vi "getOutputStateArray.vi"(8 "error in (no error)":errorcluster, 10 "configuration_name":string, 11 "HWConfiguration in":refnum<class "HWConfigurations.lvclass">) -> (0 "error out":errorcluster, 2 "outputStateArray":cluster{"channel":string, "state":string}[](array[cluster]), 3 "HWConfiguration out":refnum<class "HWConfigurations.lvclass">)   [LabVIEW 2009, in "Tools.lvlib" / "DatabaseHelpers.lvlib" / "HWConfigurations.lvclass"]
uses:
  HWConfigurations.lvclass
  HWConfigurations.lvclass/HWConfigurations.ctl
  OutputConfiguration/OutputConfiguration.lvclass
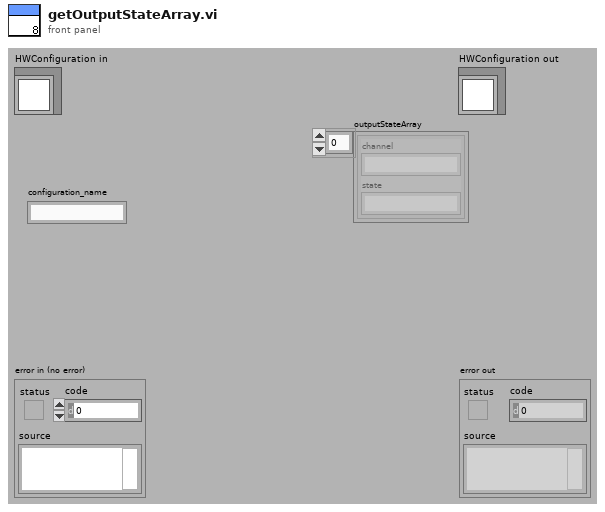
[diagram p1: front panel]
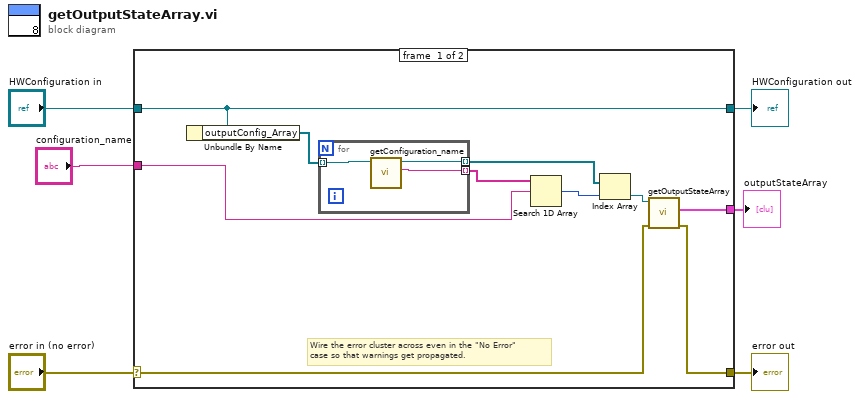
[diagram p0: block diagram]
diagram:
  n1 = case shown="No Error" "error in (no error)" {
    selector: "error in (no error)" -> [w9 w21]
    tunnel: [w8 w21] -> w5
    tunnel: [w16 w20] -> w3
    tunnel: "HWConfiguration in" -> [w16 w20]
    tunnel: "configuration_name" -> [w13 _]
    tunnel: [w7 _] -> w1
    frame #0 {
      # "Wire the error cluster across even in the \"No Error\"\ncase so that warnings get propagated."
      n2 = Unbundle By Name(w16) -> ("outputConfig_Array"=w15:refnum<class "OutputConfiguration.lvclass">[])
      n3 = for {
        tunnel: w15 -> [w19] mode=indexing
        tunnel: [w18] -> w14 mode=indexing
        tunnel: [w17] -> w12 mode=indexing
        n4 = call-dynamic "getConfiguration_name.vi"("OutputConfiguration.lvclass in"=w19) -> ("configuration_name"=w18:string, "OutputConfiguration.lvclass out"=w17:refnum<class "OutputConfiguration.lvclass">)  [unwired: 8 in, 1 out]
      }
      n5 = Search 1D Array(1D array=w14, element=w13) -> (index of element=w11:i32)  [unwired: 1 in]
      n6 = Index Array(array=w12, index=w11) -> (element=w10:refnum<class "OutputConfiguration.lvclass">)
      n7 = call "getOutputStateArray.vi"("error in (no error)"=w9, "OutputConfiguration in"=w10) -> ("error out"=w8:errorcluster, "outputStateArray"=w7:cluster{"channel":string, "state":string}[])  [unwired: 7 in, 1 out]
    }
    frame #1 {
    }
  }
  "error out" <- w5
  "HWConfiguration out" <- w3
  "outputStateArray" <- w1
